vi "Is Generated Variable.vi"(11 "String":string="v40be5e6802abc8d90698f5449fac5fb9") -> (2 "Is generated variable?":bool=TRUE, 3 "String (dup)":string="v40be5e6802abc8d90698f5449fac5fb9")   [LabVIEW 2017]
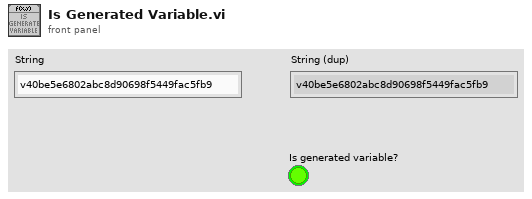
[diagram p1: front panel]
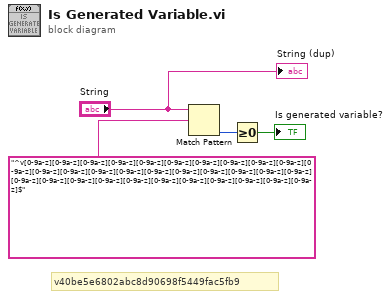
[diagram p0: block diagram]
diagram:
  # "v40be5e6802abc8d90698f5449fac5fb9"
  n1 = Match Pattern(string="String", regular expression="^v[0-9a-z][0-9a-z][0-9a-z][0-9a-z][0-9a-z][0-9a-z][0-9a-z][0-9a-z][0-9a-z][0-9a-z][0-9a-z][0-9a-z][0-9a-z][0-9a-z][0-9a-z][0-9a-z][0-9a-z][0-9a-z][0-9a-z][0-9a-z][0-9a-z][0-9a-z][0-9a-z][0-9a-z][0-9a-z][0-9a-z][0-9a-z][0-9a-z][0-9a-z][0-9a-z][0-9a-z][0-9a-z]$") -> (offset past match=w4:i32)  [unwired: 1 in, 3 out]
  n2 = Greater Or Equal To 0?(x=w4) -> (x >= 0?=→"Is generated variable?":bool)
  "String (dup)" <- "String"
